vi "Tx Bool flag set false_USRP1.vi"(3 "error in (no error)":errorcluster) -> (10 "error out":errorcluster)   [LabVIEW 2021]
uses:
  system stop.vi
panel:
  out "Time Lapse":bool
  out "before loop":timestamp
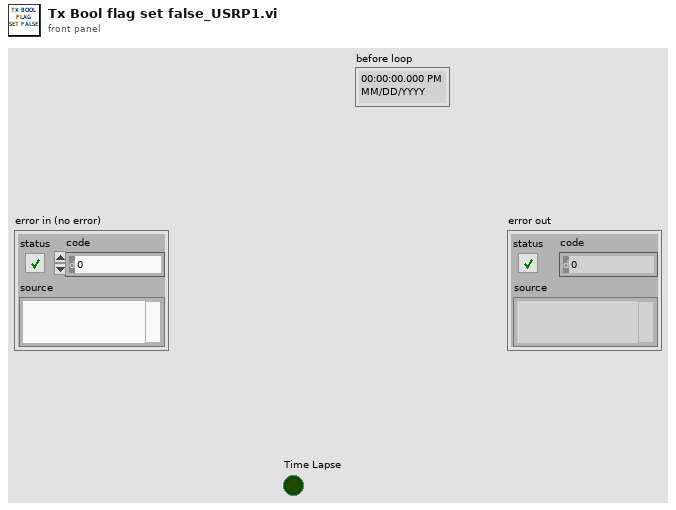
[diagram p1: front panel]
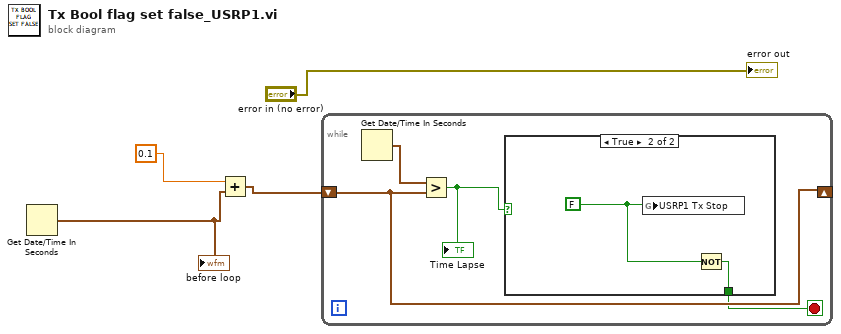
[diagram p0: block diagram]
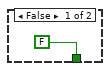
[diagram p2: hidden frame]
diagram:
  n1 = Get Date/Time In Seconds() -> (seconds since 1Jan1904=w2:timestamp)
  "before loop" <- w2
  n2 = Add(x=0.1, y=w2) -> (x+y=w1:timestamp)
  n3 = while {
    shift-right: [w7] -> _
    shift-left: w1 -> [w7]
    stop <- w6 stop-if-true
    n4 = Get Date/Time In Seconds() -> (seconds since 1Jan1904=w8:timestamp)
    n5 = Greater?(x=w8, y=w7) -> (0:w5:bool)
    "Time Lapse" <- w5
    n6 = case shown="True" w5 {
      tunnel: [FALSE w10] -> w6
      frame False {
      }
      frame True {
        w11 = FALSE
        n7 = global write "system stop.vi" "USRP1 Tx Stop"(w11) -> ()
        n8 = Not(x=w11) -> (.not. x?=w10:bool)
      }
    }
  }
  "error out" <- "error in (no error)"
